vi "MAIN_test.vi"() -> ()   [LabVIEW 2016]
uses:
  <vilib>/Utility/file.llb/Write Delimited Spreadsheet (I64).vi
  BT-Android_AE_library/BT-Android_interface.lvlib
panel:
  in  "display file path (dialog if empty)":path=path "D:/Data/intan"
  in  "display存盘":bool=TRUE
  out "35通道波形":u16[][](graph)
  in  "receive file path (dialog if empty)":path=path "D:/Data/intan"
  in  "receive存盘":bool=TRUE
  in  "receive frequence":i32=10
  in  "END CONVERT":bool
  in  "START CONVERT":bool
  out "End Character?":bool
  out "send timeout":bool=TRUE
  out "?":bool=TRUE
  in  "Channels":i32=35
  in  "Display":bool=TRUE
  in  "Send":bool
  in  "Receive":bool=TRUE
  in  "Data Send":string
  out "error out":errorcluster
  in  "Close Com":bool
  in  "Select COM before run":refnum<visa-resource-name>="COM4"
  in  "timeout (10sec)":u32=10000
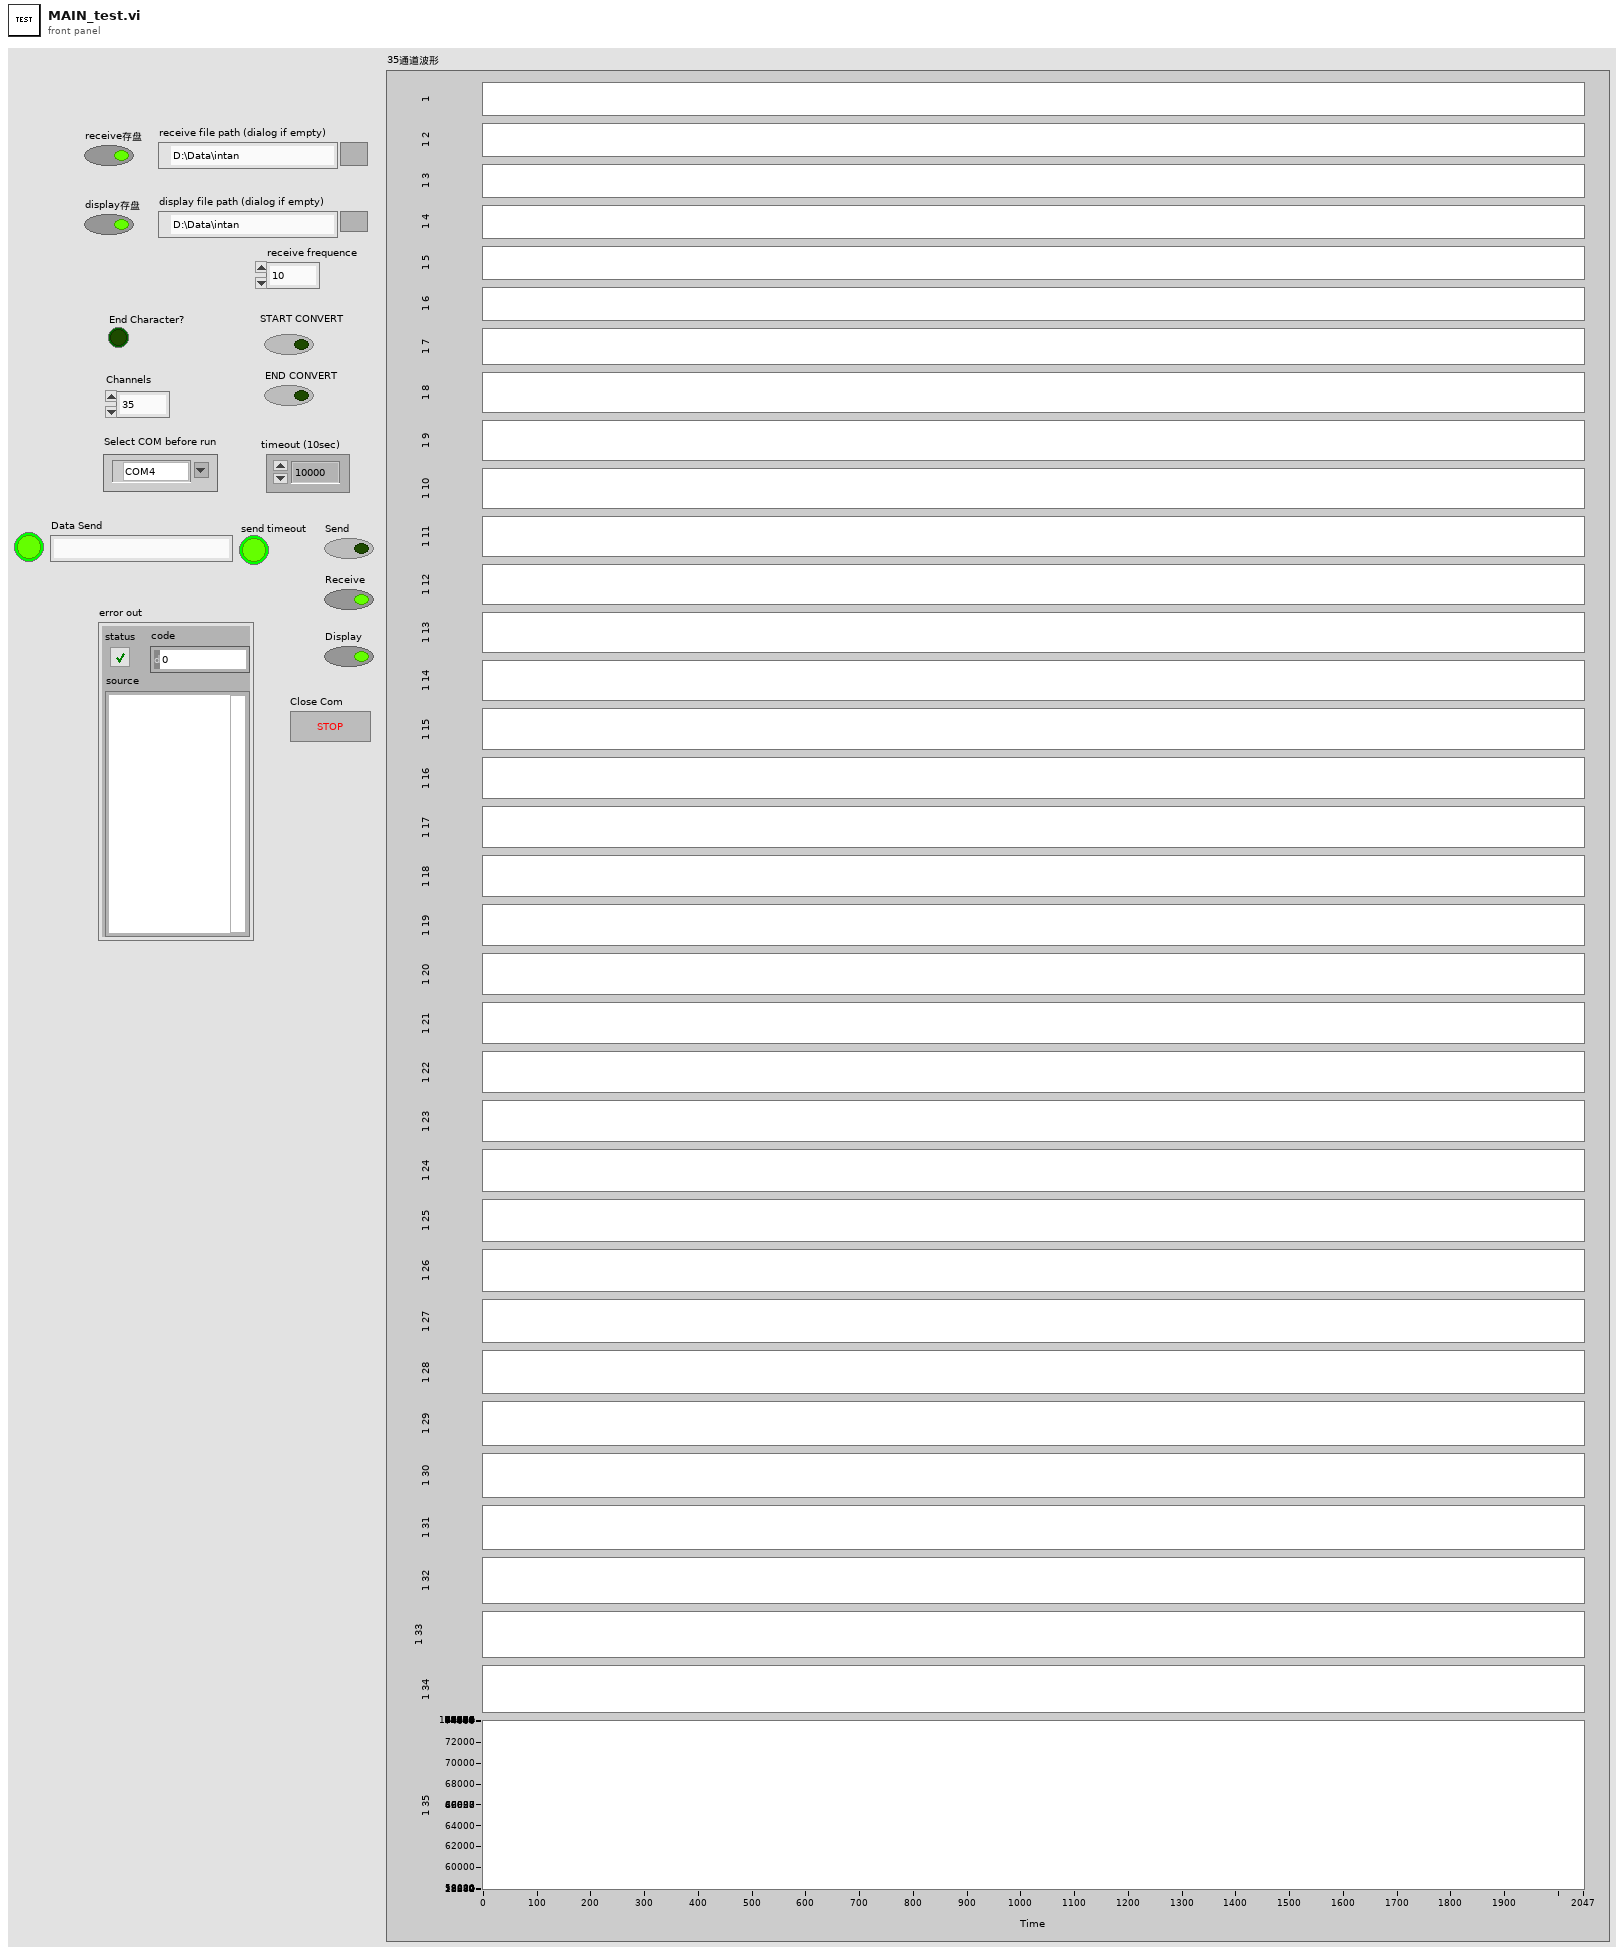
[diagram p1: front panel]
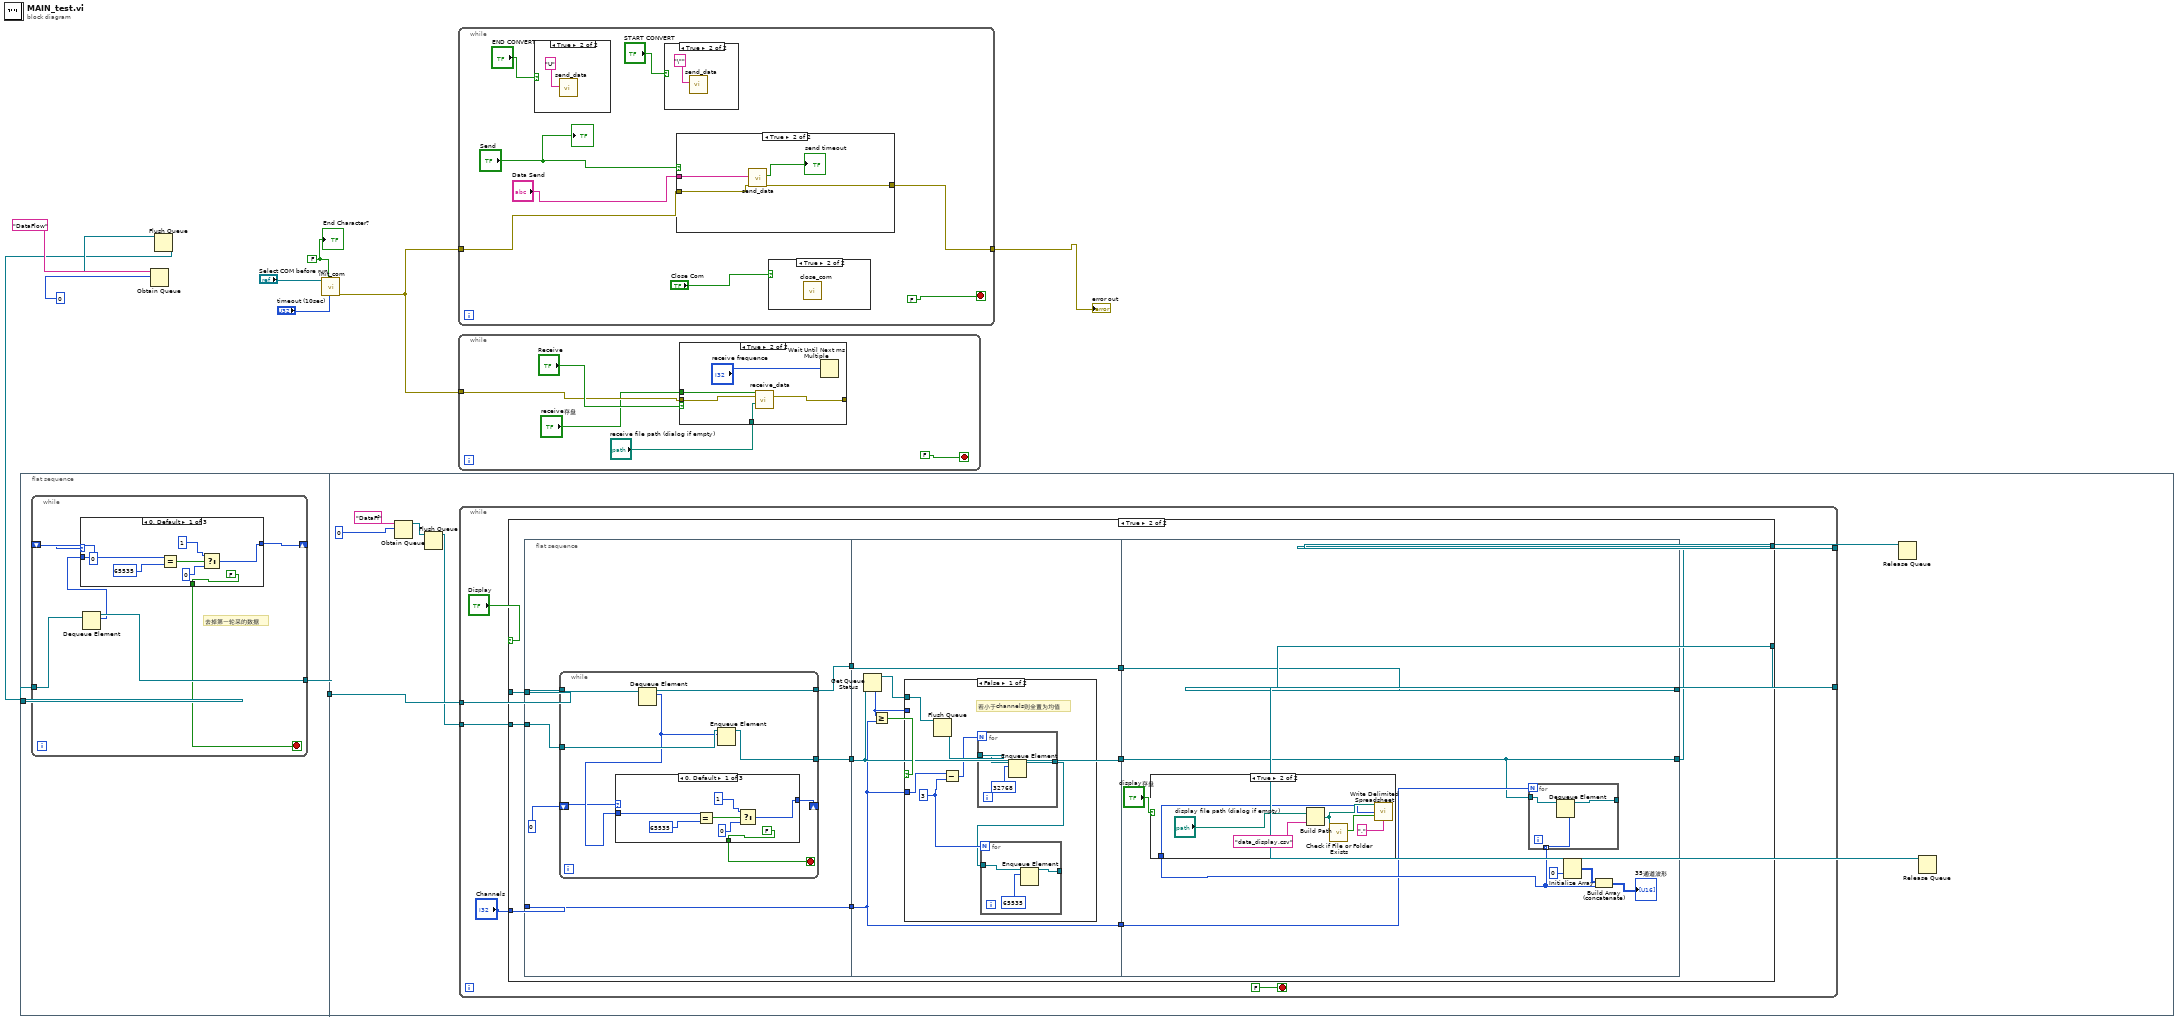
[diagram p0: block diagram]
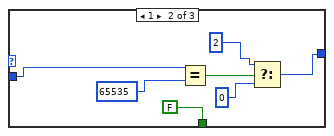
[diagram p2: hidden frame]
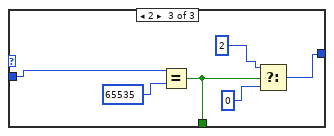
[diagram p3: hidden frame]
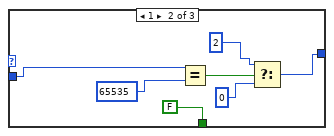
[diagram p5: hidden frame]
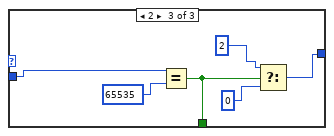
[diagram p6: hidden frame]
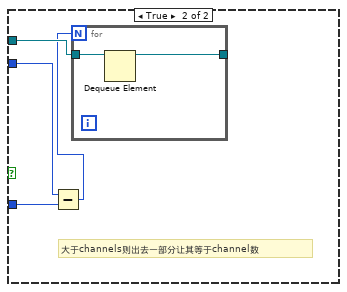
[diagram p7: hidden frame]
diagram:
  w4 = FALSE ("End Write on Termination Character?")
  n1 = flat-sequence {
    tunnel: w2 -> [w13]
    tunnel: [w12] -> w1
    tunnel: w1 -> [w45]
    frame #0 {
      n2 = while {
        tunnel: w13 -> [w19]
        tunnel: [w18] -> w12
        shift-right: [w16] -> _
        shift-left: 0 -> [w17]
        stop <- w14 stop-if-true
        # "去掉第一轮采的数据"
        n3 = Dequeue Element(queue=w19) -> (queue out=w18:refnum<queue>, element=w15:u16)  [unwired: 2 in, 2 out]
        n4 = case shown="0, Default" w17 {
          tunnel: [w21 w28 w35] -> w16
          tunnel: w15 -> [w24 w29 w36]
          tunnel: [FALSE FALSE w34] -> w14
          frame 0, Default {
            n5 = Equal?(x=w24, y=65535) -> (x = y?=w25:bool)
            n6 = Select(t=1, s=w25, f=0) -> (s? t:f=w21:i32)
          }
          frame 1 {
            n7 = Equal?(x=w29, y=65535) -> (x = y?=w32:bool)
            n8 = Select(t=2, s=w32, f=0) -> (s? t:f=w28:i32)
          }
          frame 2 {
            n9 = Equal?(x=w36, y=65535) -> (x = y?=w34:bool)
            n10 = Select(t=2, s=w34, f=0) -> (s? t:f=w35:i32)
          }
        }
      }
    }
    frame #1 {
      n11 = Obtain Queue(name (unnamed)="DataFf", element data type=u16 0) -> (queue out=w42:refnum<queue>)  [unwired: 3 in, 2 out]
      n12 = Flush Queue(queue=w42) -> (queue out=w41:refnum<queue>)  [unwired: 1 in, 2 out]
      n13 = while {
        tunnel: w45 -> [w52]
        tunnel: [w51] -> w46
        tunnel: w41 -> [w49]
        tunnel: [w47] -> w40
        stop <- FALSE ("End Write on Termination Character?") stop-if-true
        n14 = case shown="True" "Display" {
          tunnel: w52 -> [w55 w66]
          tunnel: [w55 w64] -> w51
          tunnel: w49 -> [w54 w65]
          tunnel: "Channels" -> [_ w60]
          tunnel: [w54 w56] -> w47
          frame False {
          }
          frame True {
            n15 = flat-sequence {
              tunnel: w66 -> [w72]
              tunnel: w65 -> [w71]
              tunnel: [w69] -> w63
              tunnel: [w68] -> w62
              tunnel: [w67] -> w61
              tunnel: w60 -> [w67]
              tunnel: w63 -> [w102]
              tunnel: w62 -> [w106]
              tunnel: w61 -> [w101]
              tunnel: [w102] -> w59
              tunnel: [w106] -> w58
              tunnel: [w101] -> w57
              tunnel: [w132] -> w64
              tunnel: [w125] -> w56
              tunnel: w59 -> [w125]
              tunnel: w58 -> [w132]
              tunnel: w57 -> [w126]
              frame #0 {
                n16 = while {
                  tunnel: w72 -> [w80]
                  tunnel: [w79] -> w68
                  tunnel: w71 -> [w78]
                  shift-right: [w75] -> _
                  shift-left: u16 0 -> [w76]
                  tunnel: [w73] -> w69
                  stop <- w74 stop-if-true
                  n17 = Dequeue Element(queue=w80) -> (queue out=w79:refnum<queue>, element=w77:u16)  [unwired: 2 in, 2 out]
                  n18 = case shown="0, Default" w76 {
                    tunnel: [w82 w89 w96] -> w75
                    tunnel: w77 -> [w85 w90 w97]
                    tunnel: [FALSE FALSE w95] -> w74
                    frame 0, Default {
                      n19 = Equal?(x=w85, y=65535) -> (x = y?=w86:bool)
                      n20 = Select(t=1, s=w86, f=0) -> (s? t:f=w82:i32)
                    }
                    frame 1 {
                      n21 = Equal?(x=w90, y=65535) -> (x = y?=w93:bool)
                      n22 = Select(t=2, s=w93, f=0) -> (s? t:f=w89:i32)
                    }
                    frame 2 {
                      n23 = Equal?(x=w97, y=65535) -> (x = y?=w95:bool)
                      n24 = Select(t=2, s=w95, f=0) -> (s? t:f=w96:i32)
                    }
                  }
                  n25 = Enqueue Element(queue=w78, element=w77) -> (queue out=w73:refnum<queue>)  [unwired: 2 in, 2 out]
                }
              }
              frame #1 {
                n26 = Get Queue Status(queue=w102) -> (queue out=w103:refnum<queue>, # elements in queue=w104:i32)  [unwired: 2 in, 6 out]
                n27 = Greater Or Equal?(x=w104, y=w101) -> (x >= y?=w105:bool)
                n28 = case shown="False" w105 {
                  tunnel: w103 -> [w112 w122]
                  tunnel: w104 -> [_ w121]
                  tunnel: w101 -> [w110 w120]
                  frame False {
                    w108 = 3
                    # "若小于channels则全置为均值"
                    n29 = Flush Queue(queue=w112) -> (queue out=w111:refnum<queue>)  [unwired: 1 in, 2 out]
                    n30 = Subtract(x=w110, y=w108) -> (x-y=w109:i32)
                    n31 = for {
                      N: w109 -> [_]
                      tunnel: w111 -> [w118]
                      tunnel: [w116] -> w107
                      n32 = Enqueue Element(queue=w118, element=u16 32768) -> (queue out=w116:refnum<queue>)  [unwired: 2 in, 2 out]
                    }
                    n33 = for {
                      N: w108 -> [_]
                      tunnel: w107 -> [w115]
                      tunnel: [w113] -> _
                      n34 = Enqueue Element(queue=w115, element=u16 65535) -> (queue out=w113:refnum<queue>)  [unwired: 2 in, 2 out]
                    }
                  }
                  frame True {
                    # "大于channels则出去一部分让其等于channel数"
                    n35 = Subtract(x=w121, y=w120) -> (x-y=w119:i32)
                    n36 = for {
                      N: w119 -> [_]
                      tunnel: w122 -> [w124]
                      tunnel: [w123] -> _
                      n37 = Dequeue Element(queue=w124) -> (queue out=w123:refnum<queue>)  [unwired: 2 in, 3 out]
                    }
                  }
                }
              }
              frame #2 {
                w130 = u16 0
                n38 = for {
                  N: w126 -> [_]
                  tunnel: [w135] -> w127 mode=indexing
                  tunnel: [w134] -> _
                  tunnel: w125 -> [w133]
                  n39 = Dequeue Element(queue=w133) -> (queue out=w134:refnum<queue>, element=w135:u16)  [unwired: 2 in, 2 out]
                }
                n40 = case shown="True" "display存盘" {
                  tunnel: w127 -> [_ w136]
                  frame False {
                  }
                  frame True {
                    n41 = Build Path(base path="display file path (dialog if empty)", name or relative path="data_display.csv") -> (appended path=w141:path)
                    n42 = call <vilib>:"Check if File or Folder Exists.vi"("path"=w141) -> ("file or folder exists?"=w140:bool)  [unwired: 8 in, 2 out]
                    n43 = call-poly <vilib>:"Write Delimited Spreadsheet.vi"("file path (dialog if empty)"=w141, "1D data"=w136, "append to file? (new file:F)"=w140, "delimiter (\\t)"="," ("delimiter (\\t)")) -> ()  [unwired: 10 in, 2 out]
                  }
                }
                n44 = Initialize Array(w130, w130, w130) -> (w131:u16[][])
                n45 = Build Array (concatenate)(w131, w127) -> (→"35通道波形":u16[][])
              }
            }
          }
        }
      }
      n46 = Release Queue(queue=w40) -> ()  [unwired: 2 in, 3 out]
      n47 = Release Queue(queue=w46) -> ()  [unwired: 2 in, 3 out]
    }
  }
  n48 = Obtain Queue(name (unnamed)="DataFlow", element data type=u16 0) -> (queue out=w5:refnum<queue>)  [unwired: 3 in, 2 out]
  n49 = Flush Queue(queue=w5) -> (queue out=w2:refnum<queue>)  [unwired: 1 in, 2 out]
  n50 = call "init_com.vi"("timeout (10sec)"="timeout (10sec)", "End Write on Termination Character?"=w4, "VISA resource name"="Select COM before run") -> ("error out"=w6:errorcluster)  [unwired: 8 in]
  n51 = while {
    tunnel: w6 -> [w147]
    tunnel: [w148] -> w3
    stop <- FALSE ("End Write on Termination Character?") stop-if-true
    n52 = case shown="True" "END CONVERT" {
      frame False {
      }
      frame True {
        n53 = call "send_data.vi"("send data (string)"="U" ("Data Send 2")) -> ()  [unwired: 9 in, 2 out]
      }
    }
    n54 = case shown="True" "START CONVERT" {
      frame False {
      }
      frame True {
        n55 = call "send_data.vi"("send data (string)"="\"" ("Data Send 2")) -> ()  [unwired: 9 in, 2 out]
      }
    }
    n56 = case shown="True" "Send" {
      tunnel: "Data Send" -> [_ w156]
      tunnel: w147 -> [w152 w155]
      tunnel: [w152 w154] -> w148
      frame False {
      }
      frame True {
        n57 = call "send_data.vi"("error in (no error)"=w155, "send data (string)"=w156) -> ("error out"=w154:errorcluster, "timeout?"=→"send timeout":bool)  [unwired: 8 in]
      }
    }
    n58 = case shown="True" "Close Com" {
      frame False {
      }
      frame True {
        n59 = call "close_com.vi"() -> ()  [unwired: 11 in, 1 out]
      }
    }
    "?" <- "Send"
  }
  "error out" <- w3
  n60 = while {
    tunnel: w6 -> [w160]
    stop <- FALSE ("End Write on Termination Character?") stop-if-true
    n61 = case shown="True" "Receive" {
      tunnel: w160 -> [w162 w166]
      tunnel: [w162 w165] -> _
      tunnel: "receive存盘" -> [_ w164]
      tunnel: "receive file path (dialog if empty)" -> [_ w163]
      frame False {
      }
      frame True {
        n62 = call "receive_data.vi"("存盘"=w164, "error in (no error)"=w166, "file path (dialog if empty)"=w163) -> ("error out"=w165:errorcluster)  [unwired: 11 in, 1 out]
        n63 = Wait Until Next ms Multiple(millisecond multiple="receive frequence") -> ()  [unwired: 1 out]
      }
    }
  }
  "End Character?" <- w4
